vi "Write configuration.vi"(8 "error in (no error)":errorcluster, 10 "configuration":refnum<class "CEF_serializable configuration.lvclass">, 11 "Abstract DMM in":refnum<class "FPGA Instrument.lvclass">) -> (0 "error out":errorcluster, 3 "Abstract DMM out":refnum<class "FPGA Instrument.lvclass">)   [LabVIEW 2025, in "FPGA.lvlib" / "FPGA Instrument.lvclass"]
uses:
  FPGA Instrument.lvclass
  Users/Public/Documents/Sandia National Labs/TSS Plugin/CEF.lvlibp/serializable configuration/CEF_serializable configuration.lvclass
  FPGA configuration/FPGA configuration.lvclass
  FPGA Instrument.lvclass/FPGA Instrument.ctl
panel:
  # "the child should be overrided, which inherited from serial node"
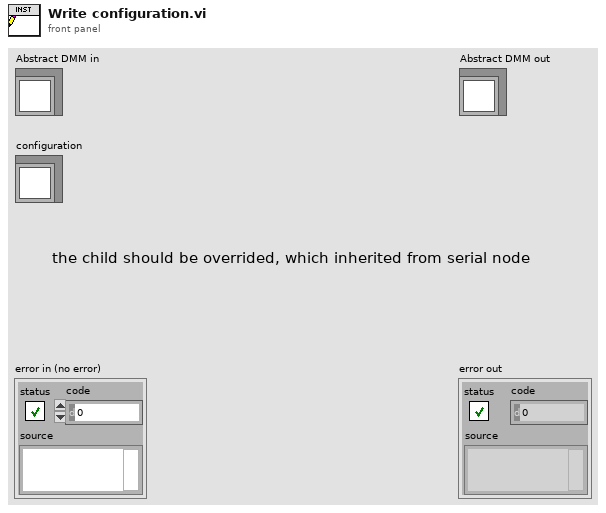
[diagram p1: front panel]
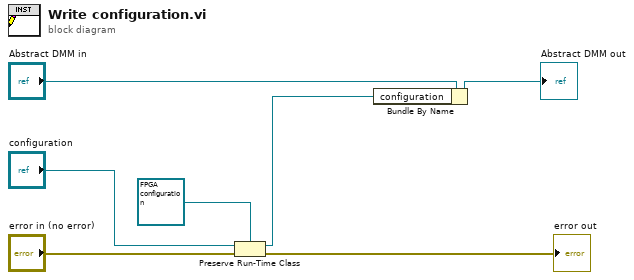
[diagram p0: block diagram]
diagram:
  n1 = Preserve Run-Time Class(object in="configuration", error in="error in (no error)", 2:refnum<class "FPGA configuration.lvclass"> refnum ("DMM.lvlib:DMM configuration.lvclass")) -> (object out=w2:refnum<class "FPGA configuration.lvclass">, error out=→"error out":errorcluster)
  n2 = Bundle By Name(cluster="Abstract DMM in", "configuration"=w2) -> (→"Abstract DMM out":refnum<class "FPGA Instrument.lvclass">)
